vi "send_trigger.vi"(8 "error in (no error)":errorcluster, 10 "trigger":T1, 11 "GenericExperiment in":refnum<class "GenericExperimentController.lvclass">) -> (0 "error out":errorcluster, 3 "GenericExperiment out":refnum<class "GenericExperimentController.lvclass">)   [LabVIEW 2010, in "GenericExperimentController.lvclass"]
uses:
  GenericExperimentController.lvclass
  trigger_enum.ctl
  common/classes/GenericToplevelComponent/GenericToplevelComponent/trigger_type_enum.ctl
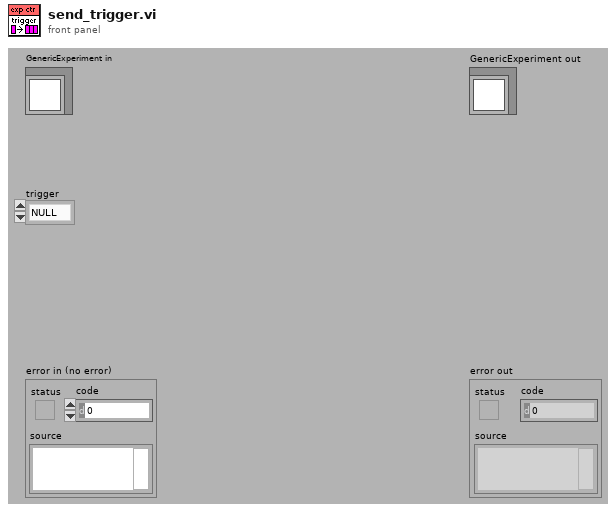
[diagram p1: front panel]
types:
  T1 = typedef "GenericExperimentController.lvclass/trigger_enum.ctl" = enum16{"NULL", "proceed", "prepare"}
  T2 = typedef "trigger_type_enum.ctl" = enum8{"external", "internal", "common"}
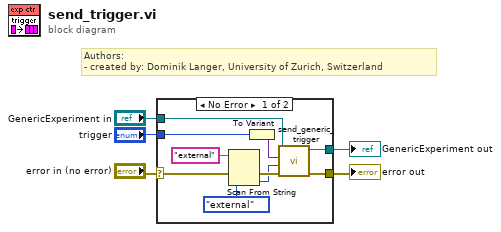
[diagram p0: block diagram]
diagram:
  # "Authors: \n- created by: Dominik Langer, University of Zurich, Switzerland"
  n1 = case shown="No Error" "error in (no error)" {
    selector: "error in (no error)" -> [w9 w17]
    tunnel: [w13 w17] -> w2
    tunnel: [w15 w16] -> w3
    tunnel: "GenericExperiment in" -> [w14 w16]
    tunnel: "trigger" -> [w12 _]
    frame No Error {
      n2 = Scan From String(input string="external", error in=w9, default 1=trigger_type_enum."external" ("trigger type")) -> (error out=w8:errorcluster, output 1=w7:T2)  [unwired: 2 in, 2 out]
      n3 = To Variant(anything=w12) -> (Variant=w11:variant)
      n4 = call-dynamic "send_generic_trigger.vi"("error in (no error)"=w8, "trigger type"=w7, "trigger variant"=w11, "GenericToplevelComponent in"=w14) -> ("error out"=w13:errorcluster, "GenericToplevelComponent out"=w15:refnum<class "GenericExperimentController.lvclass">)  [unwired: 4 in, 2 out]
    }
    frame Error {
    }
  }
  "error out" <- w2
  "GenericExperiment out" <- w3
